vi "ZControlCam1-old.vi"() -> ()   [LabVIEW 2014]
uses:
  <vilib>/vision/Vision Builder AI/API.llb/IVB Interface - VBAI Version.ctl
panel:
  in  "stop":bool
  out "Step Results":T1(array[cluster]) {"Numeric Measurement" format="%.2f"}
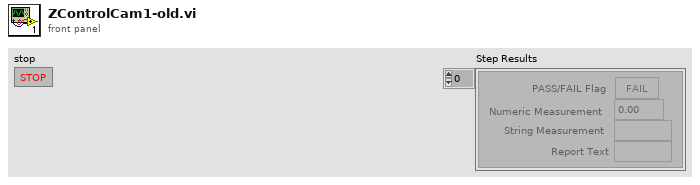
[diagram p1: front panel]
types:
  T1 = cluster{"PASS/FAIL Flag":bool, "Numeric Measurement":dbl, "String Measurement":string, "Report Text":string}[]
  T2 = typedef "IVB Interface - VBAI Version.ctl" = u16
  T3 = typedef "VBAIInterface.ctl" = refnum<k21>
  T4 = typedef "IMAQ Image.ctl" = refnum<image>
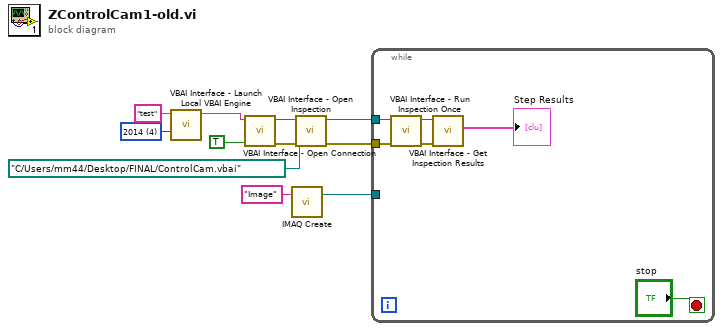
[diagram p0: block diagram]
diagram:
  w8 = T2 4 items=["2010", "2011", "2012", "2013", "2014"] ("Engine Version")
  n1 = call <vilib>:"VBAI Interface - Launch Local VBAI Engine.vi"("Engine Version"=w8, "Local VBAI Engine Name"="test") -> ("Session Name Out"=w9:string)  [unwired: 8 in, 1 out]
  n2 = call <vilib>:"VBAI Interface - Open Connection.vi"("Force Connection (False)"=TRUE, "Session In"=w9) -> ("error out"=w7:errorcluster, "Session Out"=w6:T3)  [unwired: 8 in]
  n3 = call "IMAQ Create"("Image Name"="Image") -> ("New Image"=w2:T4)  [unwired: 4 in, 1 out]
  n4 = call <vilib>:"VBAI Interface - Open Inspection.vi"("error in"=w7, "Path"=path "C:/Users/mm44/Desktop/FINAL/ControlCam.vbai", "Session In"=w6) -> ("error out"=w3:errorcluster, "Session Out"=w4:T3)  [unwired: 7 in]
  n5 = while {
    tunnel: w4 -> [w15]
    tunnel: w3 -> [w14]
    tunnel: w2 -> [_]
    stop <- "stop" stop-if-true
    n6 = call <vilib>:"VBAI Interface - Run Inspection Once.vi"("error in"=w14, "Session In"=w15) -> ("error out"=w17:errorcluster, "Session Out"=w16:T3)  [unwired: 8 in]
    n7 = call <vilib>:"VBAI Interface - Get Inspection Results.vi"("error in"=w17, "Session In"=w16) -> ("Step Results"=→"Step Results":T1)  [unwired: 3 in, 6 out]
  }
